vi "Periodic Tasks.vi"(8 "error in":errorcluster) -> ()   [LabVIEW 2015]
doc: "This VI runs in parallel to other tasks. It can contain as many user-defined periodic loops as you need. These can carry out PID or other sorts of timed response."
uses:
  <vilib>/Rock Robotics/WPI/Utilities/WPI_GetSetVariantRefNum.vi
  Robot Global Data.vi
  <vilib>/Rock Robotics/Network Tables/NT Write Boolean.vi
  <vilib>/Rock Robotics/Network Tables/NT Write Number.vi
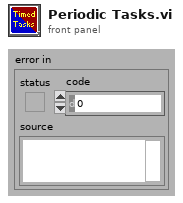
[diagram p1: front panel]
types:
  T1 = typedef "WPI_JoystickDevRef.ctl" = cluster{"Device":T2}
  T2 = typedef "WPI_JoystickDeviceEnum.ctl" = enum16{"USB 0", "USB 1", "USB 2", "USB 3", "USB 4", "USB 5"}
  T3 = typedef "WPI_RobotDriveDevRef.ctl" = cluster{"DevStatus":errorcluster, "Motors[]":T4[], "Square Inputs":bool, "Max Output":dbl}
  T4 = typedef "WPI_MotorControlDeviceRef.ctl" = cluster{"DeviceStatus":errorcluster, "Type":T5, "PWM":cluster{"PWM Channel":T6, "DeadBand":T7}, "CAN":cluster{"Device Number":u8, "Control Mode":T8, "Semaphore":T9, "Max Vout":dbl, "TalonSRX Control Mode":T10}, "Invert":bool}
  T5 = typedef "WPI_MotorControlType.ctl" = enum16{"PWM", "CAN", "CANTalonSRX"}
  T6 = typedef "FPGA_DIOPWMChannel.ctl" = enum8{"PWM 0", "PWM 1", "PWM 2", "PWM 3", "PWM 4", "PWM 5", "PWM 6", "PWM 7", "PWM 8", "PWM 9", "PWM MXP 0", "PWM MXP 1", "PWM MXP 2", "PWM MXP 3", "PWM MXP 4", "PWM MXP 5", "PWM MXP 6", "PWM MXP 7", "PWM MXP 8", "PWM MXP 9", "Invalid"}
  T7 = typedef "WPI_PWMDeadband.ctl" = cluster{"Name":string, "maxPositivePwm":i32, "minPositivePwm":i32, "centerPwm":i32, "maxNegativePwm":i32, "minNegativePwm":i32, "angularRange":u16}
  T8 = typedef "WPI_CANJaguar_ControlMode.ctl" = enum8{"Percent VBus", "Current", "Speed", "Position", "Voltage"}
  T9 = typedef "Semaphore RefNum" = refnum<k1>
  T10 = typedef "WPI_CANTalonSRX_APIControlMode.ctl" = enum8{"Percent VBus", "Speed", "Position", "Slave", "Unchanged / Invalid", "Voltage Compensation", "Current", "Motion Profile"}
  T11 = typedef "WPI_AccelerometerDevRef.ctl" = cluster{"DevStatus":errorcluster, "Scaling":T12, "Analog Channels":T13, "I2C Bus":T15, "SPI Bus":T16, "Accel Range":T17, "ADXL Axes":T18, "Handle":i32, "Device Address":u8, "Accel Type":enum16{"Analog", "ADXL345 I2C", "ADXL345 SPI", "Internal", "ADXL362 SPI"}}
  T12 = typedef "WPI_AccelerometerScaling.ctl" = cluster{"Gain (VoltsPerG)":dbl, "Center Voltage":dbl}
  T13 = typedef "WPI_AccelerometerAnalogChannels.ctl" = cluster{"X-Axis":T14, "Y-Axis":T14, "Z-Axis":T14}
  T14 = typedef "FPGA_AIChannel.ctl" = enum8{"AI 0", "AI 1", "AI 2", "AI 3", "AI MXP 0", "AI MXP 1", "AI MXP 2", "AI MXP 3", "Invalid"}
  T15 = typedef "i2c_bus.ctl" = enum16{"I2C On-Board", "I2C MXP", "Invalid"}
  T16 = typedef "spi_bus.ctl" = enum16{"SPI On-Board, CS0", "SPI On-Board, CS1", "SPI On-Board, CS2", "SPI On-Board, CS3", "SPI MXP", "Invalid"}
  T17 = typedef "ADXL345 Range.ctl" = u8
  T18 = typedef "WPI_AccelerometerADXL345 Axes.ctl" = cluster{"X-Axis":bool, "Y-Axis":bool, "Z-Axis":bool}
  T19 = cluster{"JoystickDevRef":T1, "RobotDriveDevRef":T3}
  T20 = typedef "WPI_GyroDevRef.ctl" = cluster{"DevStatus":errorcluster, "Analog Channel":T14, "Offset":dbl, "Gain (VoltsPerDegree/Second)":dbl, "Gyro Type":enum16{"Analog", "XRS450"}, "Handle":i32, "SPI Bus":T16, "Device Found":bool, "Sample Rate":dbl, "Calibrate On Open":bool}
  T21 = cluster{"X-Axis":dbl, "Y-Axis":dbl, "Z-Axis":dbl}
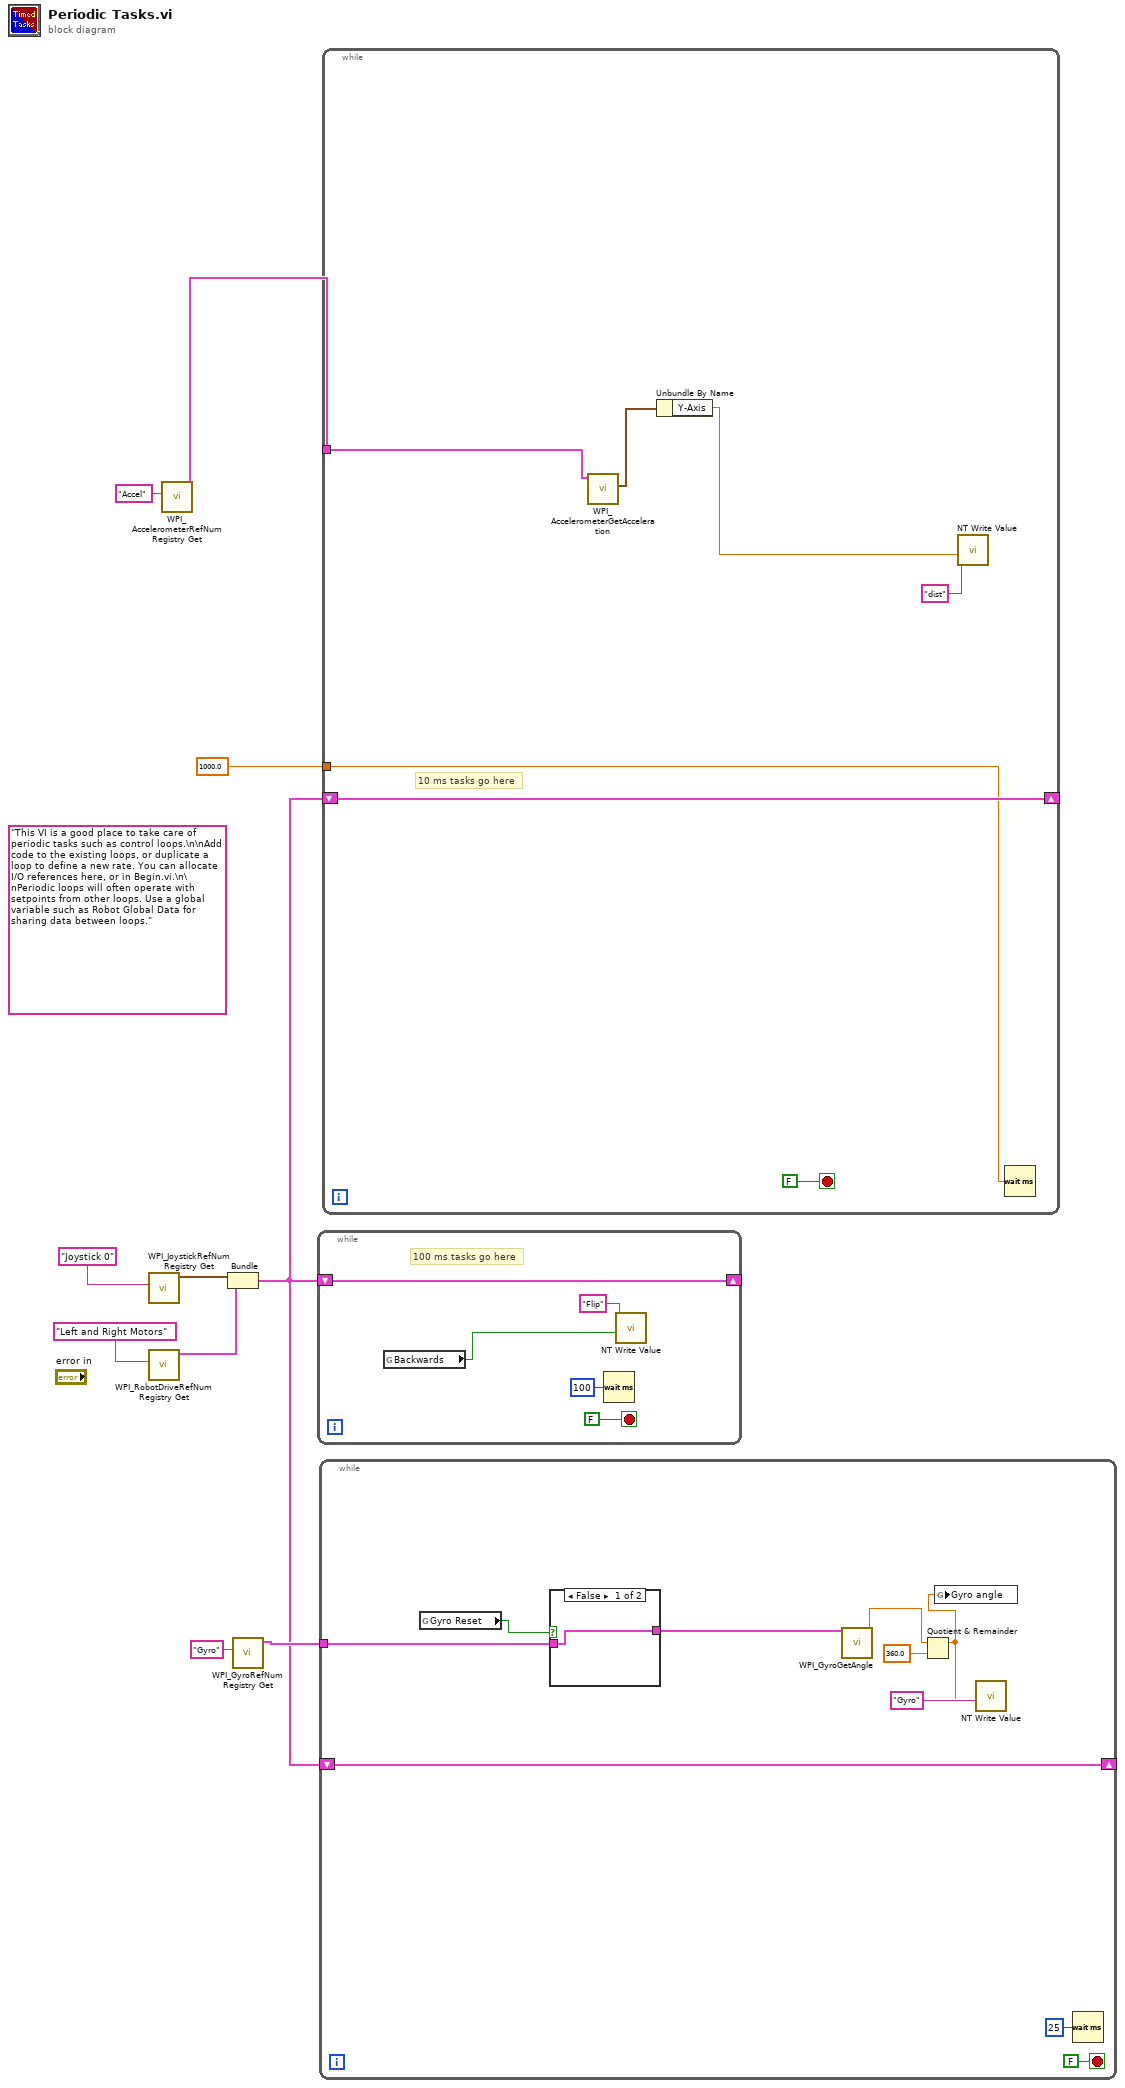
[diagram p0: block diagram]
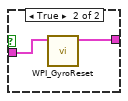
[diagram p2: hidden frame]
diagram:
  (unwired) "This VI is a good place to take care of periodic tasks such as control loops.\n\nAdd code to the existing loops, or duplicate a loop to define a new rate. You can allocate I/O references here, or in Begin.vi.\n\nPeriodic loops will often operate with setpoints from other loops. Use a global variable such as Robot Global Data for sharing data between loops."
  n1 = call <vilib>:"WPI_JoystickRefNum Registry Get.vi"("refnum name"="Joystick 0") -> ("JoystickDevRef"=w8:T1)  [unwired: 1 in, 9 out]
  n2 = call <vilib>:"WPI_RobotDriveRefNum Registry Get.vi"("refnum name"="Left and Right Motors") -> ("RobotDriveDevRef"=w7:T3)  [unwired: 1 in, 9 out]
  n3 = call <vilib>:"WPI_AccelerometerRefNum Registry Get.vi"("refnum name"="Accel") -> ("AccelerometerDevRef"=w5:T11)  [unwired: 9 in, 1 out]
  n4 = Bundle("JoystickDevRef"=w8, "RobotDriveDevRef"=w7) -> (w1:T19)  [unwired: 1 out]
  n5 = call <vilib>:"WPI_GyroRefNum Registry Get.vi"("refnum name"="Gyro") -> ("GyroDevRef"=w3:T20)  [unwired: 9 in, 1 out]
  n6 = while {
    shift-right: [w13] -> _
    shift-left: w1 -> [w13]
    stop <- FALSE stop-if-true
    # "100 ms tasks go here"
    n7 = global read "Robot Global Data.vi" "Backwards"() -> (w12:bool)
    n8 = Wait (ms)(milliseconds to wait=u32 100) -> ()  [unwired: 1 out]
    n9 = call-poly <vilib>:"NT Write Value.vi"("Boolean"=w12, "Name"="Flip") -> ()  [unwired: 9 in, 1 out]
  }
  n10 = while {
    tunnel: w3 -> [w19]
    shift-right: [w18] -> _
    shift-left: w1 -> [w18]
    stop <- FALSE stop-if-true
    n11 = global read "Robot Global Data.vi" "Gyro Reset"() -> (w22:bool)
    n12 = case shown="False" w22 {
      tunnel: [w26 w28] -> w21
      tunnel: w19 -> [w26 w27]
      frame False {
      }
      frame True {
        n13 = call <vilib>:"WPI_GyroReset.vi"("GyroDevRef"=w27) -> ("GyroDevRef"=w28:T20)  [unwired: 9 in, 1 out]
      }
    }
    n14 = call <vilib>:"WPI_GyroGetAngle.vi"("GyroDevRef"=w21) -> ("Angle"=w17:dbl)  [unwired: 6 in, 4 out]
    n15 = Quotient & Remainder(x=w17, y=360.0) -> (x-y*floor(x/y)=w16:dbl)  [unwired: 1 out]
    n16 = global write "Robot Global Data.vi" "Gyro angle"(w16) -> ()
    n17 = call-poly <vilib>:"NT Write Value.vi"("Numeric"=w16, "Name"="Gyro") -> ()  [unwired: 9 in, 1 out]
    n18 = Wait (ms)(milliseconds to wait=u32 25) -> ()  [unwired: 1 out]
  }
  n19 = while {
    shift-right: [w34] -> _
    shift-left: w1 -> [w34]
    tunnel: w5 -> [w33]
    tunnel: 1000.0 ("milliseconds to wait") -> [w31]
    stop <- FALSE stop-if-true
    # "10 ms tasks go here"
    n20 = call <vilib>:"WPI_AccelerometerGetAcceleration.vi"("AccelerometerDevRef"=w33) -> ("Accelerations"=w32:T21)  [unwired: 8 in, 2 out]
    n21 = Unbundle By Name(w32) -> ("Y-Axis"=w29:dbl)
    n22 = call-poly <vilib>:"NT Write Value.vi"("Numeric"=w29, "Name"="dist") -> ()  [unwired: 9 in, 1 out]
    n23 = Wait (ms)(milliseconds to wait=w31) -> ()  [unwired: 1 out]
  }
